vi "Unbenannt 1.vi"() -> ()   [LabVIEW 2020, in "FT-IR.lvlib" / "Spanfaktor.lvlib"]
uses:
  Spanfaktor.lvlib
  Sprachverwaltung/Sprachverwaltung.lvlib
  Sprachverwaltung/FGV Aktion Tabelle zerlegen.ctl
panel:
  out "Teil-String":string
  out "Tabellen-String":string
  out "Average":i32
  in  "Average:":refnum<vi>
  in  "Average:":i32=60
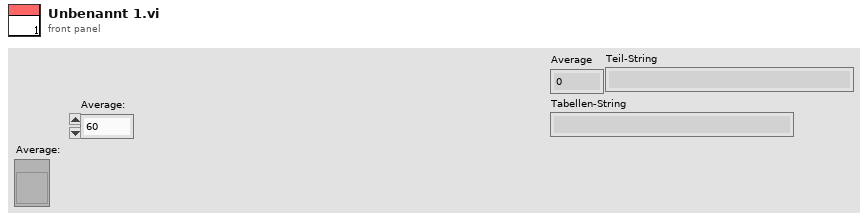
[diagram p1: front panel]
types:
  T1 = typedef "Sprachverwaltung.lvlib/FGV Aktion Tabelle zerlegen.ctl" = enum16{"laden", "vereinzeln", "speichern"}
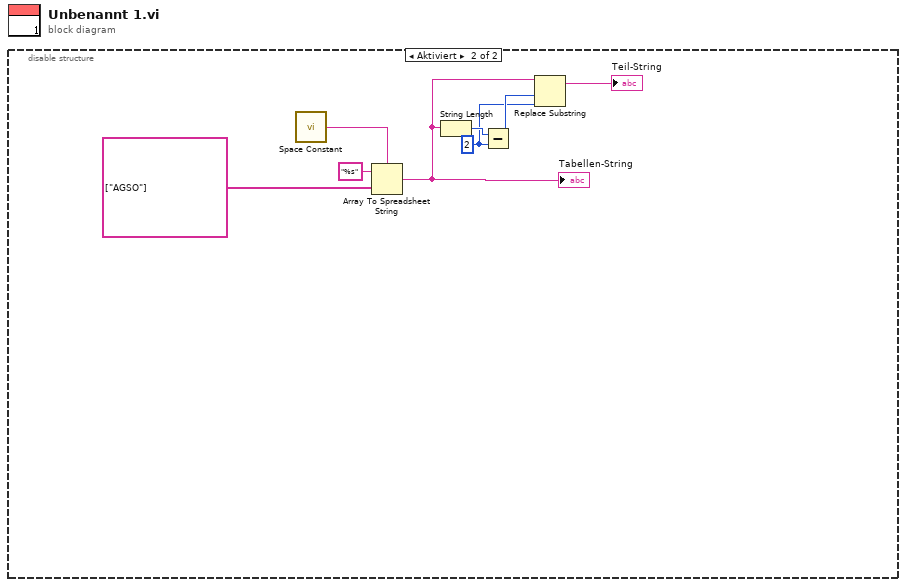
[diagram p0: block diagram]
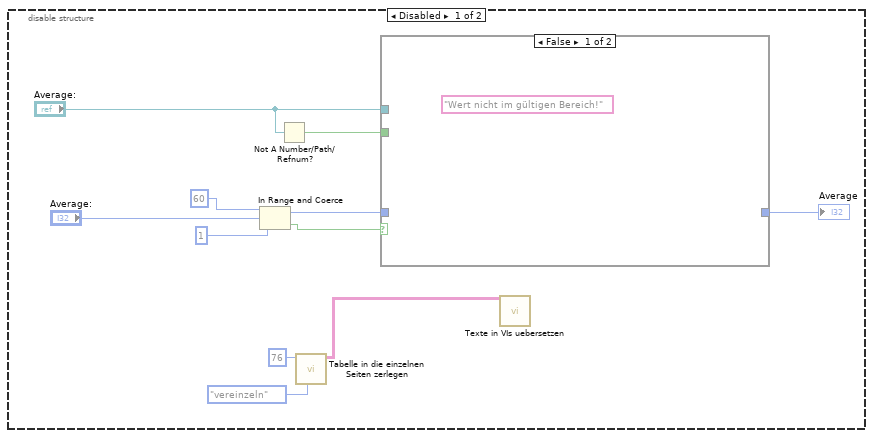
[diagram p2: hidden frame]
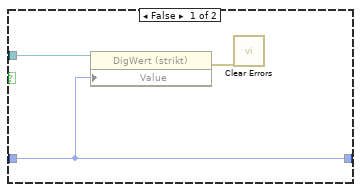
[diagram p4: hidden frame]
diagram:
  n1 = disable-structure shown="Aktiviert" {
    frame Disabled {
      n2 = In Range and Coerce(upper limit=60 ("Average over:"), x="Average:", lower limit=1 ("Average over:")) -> (coerced(x)=w6:i32, In Range?=w1:bool)
      n3 = Not A Number/Path/Refnum?(number/path/refnum="Average:") -> (NaN/Path/Refnum?=w3:bool)
      n4 = call "Tabelle in die einzelnen Seiten zerlegen.vi"("Aktion"=FGV_Aktion_Tabelle_zerlegen."vereinzeln", "Index (Seite)"=76) -> ("Sprachliste"=w5:string[][])  [unwired: 7 in, 2 out]
      n5 = case shown="False" w1 {
        tunnel: w6 -> [_ w15]
        tunnel: "Average:" -> [_ w14]
        tunnel: w3 -> [_ w13]
        tunnel: [_ w12] -> w2
        frame False {
          (unwired) "Wert nicht im gültigen Bereich!"
        }
        frame True {
          n6 = case shown="True" w13 {
            tunnel: w14 -> [w18 _]
            tunnel: w15 -> [w17 w19]
            tunnel: [w17 w19] -> w12
            frame False {
              n7 = property class="DigWert (strikt)"(reference=w18, "Value"=w17) -> (error out=w16:errorcluster)  [unwired: 1 in, 1 out]
              n8 = call <vilib>:"Clear Errors.vi"("error in (no error)"=w16) -> ()  [unwired: 5 in, 2 out]
            }
            frame True {
            }
          }
        }
      }
      "Average" <- w2
      n9 = call "Texte in VIs uebersetzen.vi"("Sprachliste"=w5) -> ()  [unwired: 10 in, 5 out]
    }
    frame Enabled {
      w21 = 2 ("y")
      n10 = call <vilib>:"Space Constant.vi"() -> ("String"=w25:string)
      n11 = Array To Spreadsheet String(delimiter (Tab)=w25, array=string[] ["AGSO"], 3:"%s" ("Format-String")) -> (spreadsheet string=w23:string)
      "Tabellen-String" <- w23
      n12 = String Length(string=w23) -> (length=w24:i32)
      n13 = Subtract(x=w24, y=w21) -> (x-y=w22:i32)
      n14 = Replace Substring(2:w21, 3:w22, 5:w23) -> (1:→"Teil-String":string)  [unwired: 1 in, 1 out]
    }
  }
